vi "Waveform Chart, Autoscale X and Y.vi"(8 "error in":errorcluster, 11 "WFGraph ref":refnum<vi>) -> (0 "error out":errorcluster, 3 "WFGraph ref dup":refnum<vi>)   [LabVIEW 2010]
doc: "This function sets the x-axis and y-axis to autoscale."
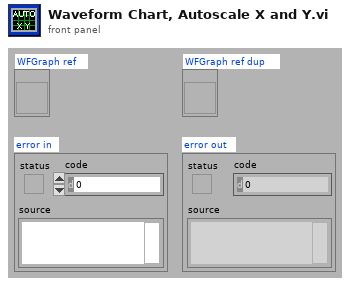
[diagram p1: front panel]
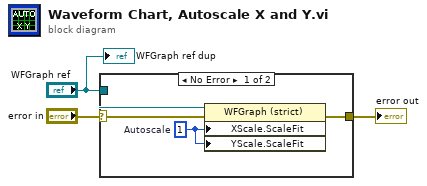
[diagram p0: block diagram]
diagram:
  n1 = case shown="No Error" "error in" {
    selector: "error in" -> [w5 w8]
    tunnel: [w7 w8] -> w2
    tunnel: "WFGraph ref" -> [w4 _]
    frame No Error {
      w6 = u8 1  # Autoscale
      n2 = property class="WFGraph (strict)"(reference=w4, error in=w5, "XScale.ScaleFit"=w6, "YScale.ScaleFit"=w6) -> (error out=w7:errorcluster)  [unwired: 1 out]
    }
    frame Error {
    }
  }
  "error out" <- w2
  "WFGraph ref dup" <- "WFGraph ref"
